vi "Log_Calagem.vi"(3 "Desloc DEC":dbl, 4 "Desloc RA":dbl, 5 "File Name":string) -> ()   [LabVIEW 2018]
panel:
  out "date string":string
  out "String":string
  out "Comando":string
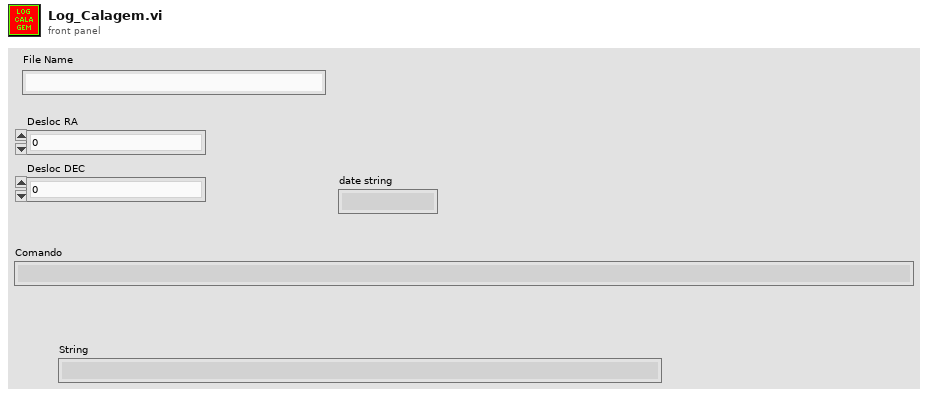
[diagram p1: front panel]
types:
  T1 = enum16{"open", "open or create", "create or replace", "create"}
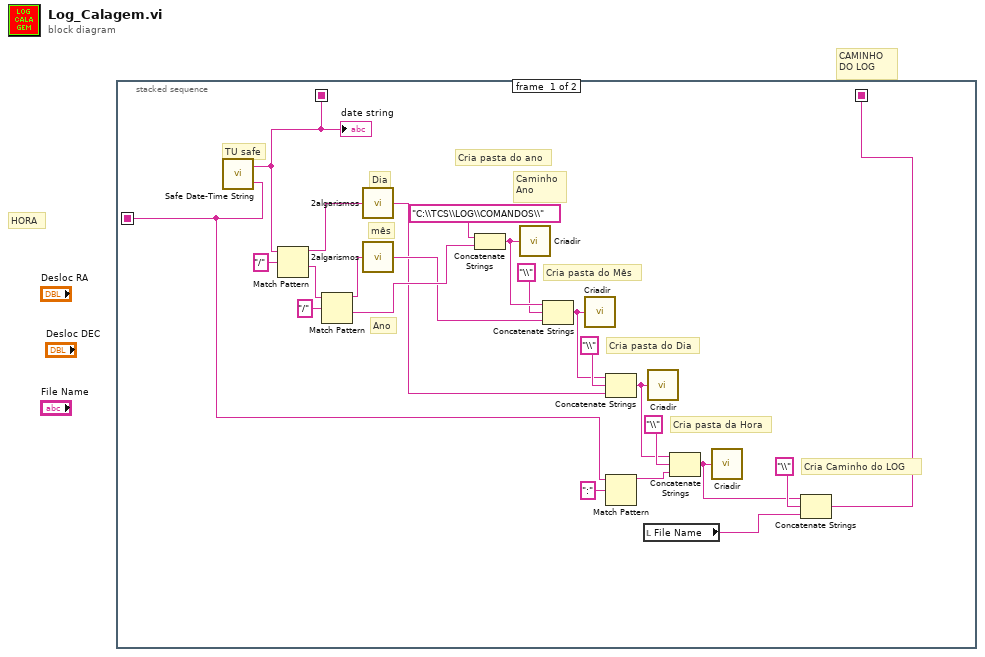
[diagram p0: block diagram]
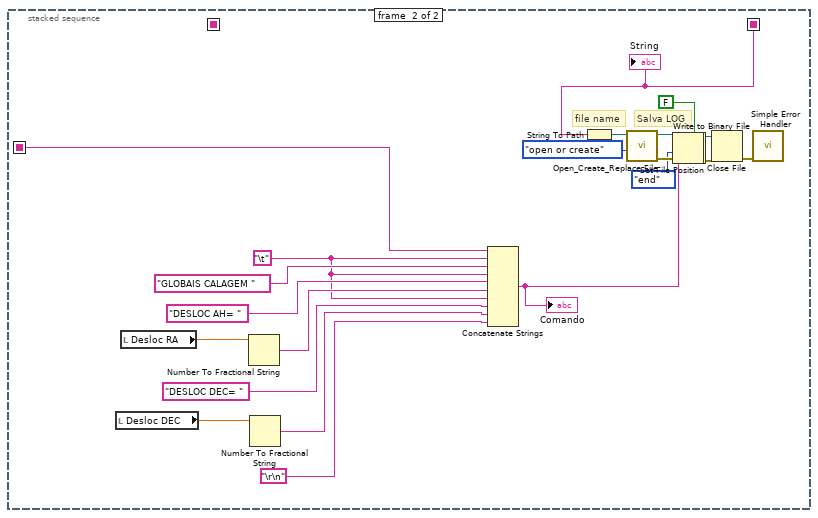
[diagram p2: hidden frame]
diagram:
  # "HORA"
  # "CAMINHO\nDO LOG"
  n1 = stacked-sequence {
    seq-local: [w9 _] -> [_ w45]
    seq-local: [w1 _] -> [_ w44]
    seq-local: [w2 _] -> [_ _]
    frame #0 {
      # "TU safe"
      # "Cria pasta da Hora"
      # "Cria Caminho do LOG"
      # "Cria pasta do Dia"
      # "Cria pasta do Mês"
      # "Caminho\nAno"
      # "Ano"
      # "mês"
      # "Dia"
      # "Cria pasta do ano"
      n2 = call "Safe Date-Time String.vi"() -> ("Safe time string"=w1:string, "Safe date string"=w2:string)  [unwired: 3 in]
      "date string" <- w2
      n3 = Match Pattern(string=w2, regular expression="/") -> (before substring=w20:string, after substring=w21:string)  [unwired: 1 in, 2 out]
      n4 = Match Pattern(string=w21, regular expression="/") -> (before substring=w19:string, after substring=w17:string)  [unwired: 1 in, 2 out]
      n5 = call "2algarismos.vi"("entrada"=w20) -> ("saida"=w11:string)
      n6 = call "2algarismos.vi"("entrada"=w19) -> ("saida"=w14:string)
      n7 = Concatenate Strings("C:\\TCS\\LOG\\COMANDOS\\" ("SOMENTE DIRETORIO"), w17) -> (w16:string)
      n8 = call "Criadir.vi"("SOMENTE DIRETORIO"=w16) -> ()  [unwired: 2 out]
      n9 = Concatenate Strings(w16, "\\" ("regular expression"), w14) -> (w12:string)
      n10 = call "Criadir.vi"("SOMENTE DIRETORIO"=w12) -> ()  [unwired: 2 out]
      n11 = Concatenate Strings(w12, "\\" ("regular expression"), w11) -> (w7:string)
      n12 = Match Pattern(string=w1, regular expression=":") -> (before substring=w5:string)  [unwired: 1 in, 3 out]
      n13 = local read "File Name"() -> (w3:string)
      n14 = call "Criadir.vi"("SOMENTE DIRETORIO"=w7) -> ()  [unwired: 2 out]
      n15 = Concatenate Strings(w7, "\\" ("regular expression"), w5) -> (w4:string)
      n16 = call "Criadir.vi"("SOMENTE DIRETORIO"=w4) -> ()  [unwired: 2 out]
      n17 = Concatenate Strings(w4, "\\" ("regular expression"), w3) -> (w9:string)
    }
    frame #1 {
      w29 = "\t"
      # "Salva LOG"
      # "file name"
      n18 = local read "Desloc DEC"() -> (w24:dbl)
      n19 = local read "Desloc RA"() -> (w25:dbl)
      n20 = Number To Fractional String(number=w25) -> (F-format string=w30:string)  [unwired: 3 in]
      n21 = Number To Fractional String(number=w24) -> (F-format string=w27:string)  [unwired: 3 in]
      n22 = Concatenate Strings(w44, w29, "GLOBAIS CALAGEM " ("date string"), w29, "DESLOC AH= " ("date string"), w30, w29, "DESLOC DEC= " ("date string"), w27, "\r\n") -> (w46:string)
      "Comando" <- w46
      n23 = String To Path(string=w45) -> (path=w36:path)
      n24 = call <vilib>:"Open_Create_Replace File.vi"("function (open:0)"=T1."open or create", "file path"=w36) -> ("error out"=w39:errorcluster, "refnum"=w42:refnum<file>)  [unwired: 6 in, 2 out]
      n25 = Set File Position(refnum=w42, from (0:start)=enum16{"start", "end", "current"}."end" ("pos mode (0:2)"), error in=w39) -> (refnum out=w35:refnum<file>, error out=w34:errorcluster)  [unwired: 1 in]
      n26 = Write to Binary File(file (use dialog)=w35, data=w46, error in=w34, 5:FALSE ("prepend array or string size? (T)")) -> (refnum out=w41:refnum<file>, error out=w40:errorcluster)  [unwired: 2 in, 1 out]
      n27 = Close File(refnum=w41, error in=w40) -> (error out=w43:errorcluster)  [unwired: 1 out]
      n28 = call <vilib>:"Simple Error Handler.vi"("error in (no error)"=w43) -> ()  [unwired: 4 in, 5 out]
      "String" <- w45
    }
  }
